vi "Register Hamburger Menu VI.vi"(8 "error in (no error)":errorcluster, 10 "Hamburger Support Control Refnum":refnum<vi>, 11 "HamburgerMenu Obj in":refnum<class "HamburgerMenu.lvclass">) -> (0 "error out":errorcluster, 3 "HamburgerMenu Obj":refnum<class "HamburgerMenu.lvclass">)   [LabVIEW 2017, in "Hamburger Menu Library.lvlib" / "HamburgerMenu.lvclass"]
uses:
  HamburgerMenu.lvclass
  HamburgerMenu.lvclass/HamburgerMenu.ctl
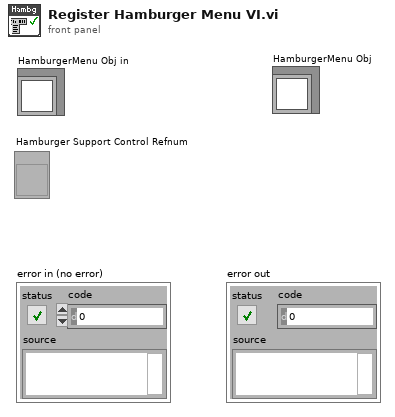
[diagram p1: front panel]
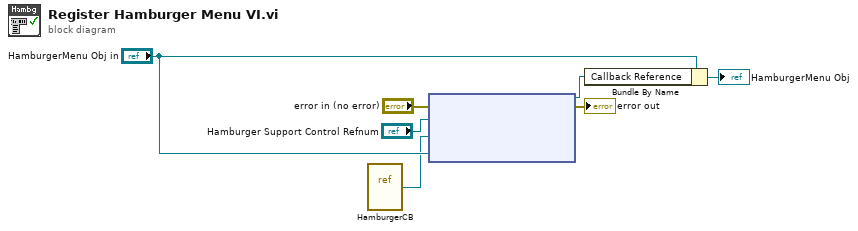
[diagram p0: block diagram]
diagram:
  n1 = vi-ref "HamburgerCB.vi"() -> (w1:refnum<vi>)
  n2 = node("error in (no error)", "Hamburger Support Control Refnum", w1, "HamburgerMenu Obj in") -> (w4:refnum<k27>, →"error out":errorcluster)  [unwired: 1 in]
  n3 = Bundle By Name(cluster="HamburgerMenu Obj in", "Callback Reference"=w4) -> (→"HamburgerMenu Obj":refnum<class "HamburgerMenu.lvclass">)
